vi "read_heater_needle-valve.vi"(0 "refnum":refnum<file>) -> ()   [LabVIEW 2016]
uses:
  Instrument_Setup.vi
  Global/Global Variables/Data_Display_global.vi
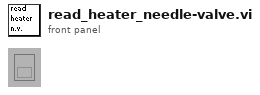
[diagram p1: front panel]
types:
  T1 = typedef "20TVTI_Cluster.ctl" = cluster{"Temperatur (K)":dbl, "Setpoint (K)":dbl, "Rate (K/min)":dbl, "Heater (%)":dbl, "NV (%)":dbl, "Heater Manual":bool, "NV Manual":bool, "Go to Set":bool, "Pressure":dbl, "Heater SP":dbl, "Valid?":bool, "Set Heater SP":bool, "Set NV SP":bool, "Heater (%) Display":dbl, "NV (%) Display":dbl, "NV Setpoint":dbl, "Change Heater Status":bool, "Change NV Status":bool, "Change Sweep Type":bool}
  T2 = typedef "VTI-cluster.ctl" = cluster{"Temperatur (K)":dbl, "Setpoint (K)":dbl, "Rate (K/min)":dbl, "Heater (%)":dbl, "NV (%)":dbl, "Heater Manual":bool, "NV Manual":bool, "Go to Set":bool, "Pressure":dbl, "Heater SP":dbl, "Valid?":bool, "Set Heater SP":bool, "Set NV SP":bool, "Heater (%) Display":dbl, "NV (%) Display":dbl, "NV Setpoint":dbl, "Change Heater Status":bool, "Change NV Status":bool, "Sample 3":dbl, "Sample 2":dbl, "Sweep-State":bool, "Set Auto PID":bool, "Auto PID":bool, "Stopp":bool, "Setpoint-Sweep":dbl}
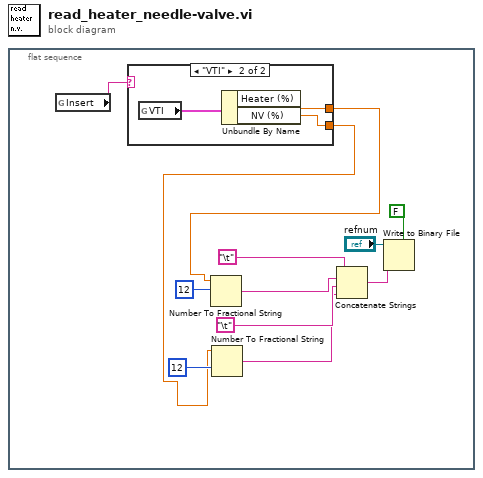
[diagram p0: block diagram]
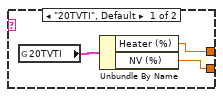
[diagram p2: hidden frame]
diagram:
  n1 = flat-sequence {
    frame #0 {
      n2 = global read "Instrument_Setup.vi" "Insert"() -> (w3:string)
      n3 = case shown="\"VTI\"" w3 {
        tunnel: [w14 w18] -> w2
        tunnel: [w13 w17] -> w1
        frame "20TVTI", Default {
          n4 = global read "Data_Display_global.vi" "20TVTI"() -> (w15:T1)
          n5 = Unbundle By Name(w15) -> ("Heater (%)"=w14:dbl, "NV (%)"=w13:dbl)
        }
        frame "VTI" {
          n6 = global read "Data_Display_global.vi" "VTI"() -> (w16:T2)
          n7 = Unbundle By Name(w16) -> ("Heater (%)"=w18:dbl, "NV (%)"=w17:dbl)
        }
      }
      n8 = Number To Fractional String(number=w2, precision (6)=i16 12) -> (F-format string=w7:string)  [unwired: 2 in]
      n9 = Number To Fractional String(number=w1, precision (6)=i16 12) -> (F-format string=w8:string)  [unwired: 2 in]
      n10 = Concatenate Strings("\t", w7, "\t", w8) -> (w5:string)
      n11 = Write to Binary File ("Write File")(file (use dialog)="refnum", data=w5, 5:FALSE ("prepend array or string size? (T)")) -> ()  [unwired: 3 in, 3 out]
    }
  }
